vi "Set Dialog Properties.vi"(8 "error in (no error)":errorcluster, 10 "Boolean":bool, 11 "VI in":refnum<vi>) -> (0 "error out":errorcluster, 2 "VI out":refnum<vi>)   [LabVIEW 2015]
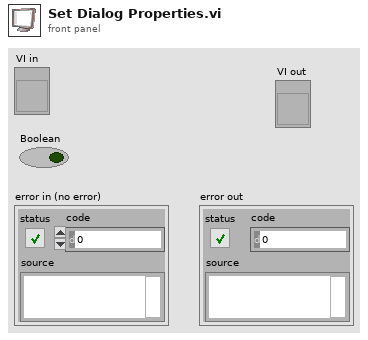
[diagram p1: front panel]
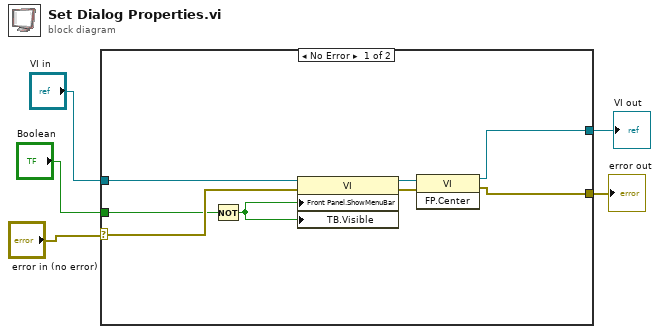
[diagram p0: block diagram]
diagram:
  n1 = case shown="No Error" "error in (no error)" {
    selector: "error in (no error)" -> [w11 w14]
    tunnel: [w10 w14] -> w4
    tunnel: "Boolean" -> [w9 _]
    tunnel: "VI in" -> [w7 w15]
    tunnel: [w6 w15] -> w1
    frame No Error {
      n2 = Not(x=w9) -> (.not. x?=w8:bool)
      n3 = property class="VI"(reference=w7, error in=w11, "Front Panel.ShowMenuBar"=w8, "TB.Visible"=w8) -> (reference out=w13:refnum<vi>, error out=w12:errorcluster)
      n4 = invoke class="VI" method="FP.Center"(reference=w13, error in=w12) -> (reference out=w6:refnum<vi>, error out=w10:errorcluster)  [unwired: 1 in, 1 out]
    }
    frame Error {
    }
  }
  "error out" <- w4
  "VI out" <- w1
